vi "Commutator_close.vi"(1 "VISA in":T1) -> (0 "Error out":errorcluster)   [LabVIEW 2011]
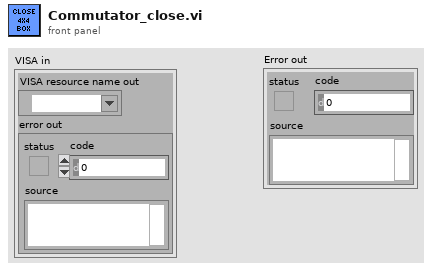
[diagram p1: front panel]
types:
  T1 = cluster{"VISA resource name out":refnum<visa-resource-name>, "error out":errorcluster}
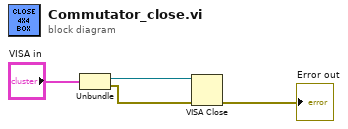
[diagram p0: block diagram]
diagram:
  n1 = Unbundle("VISA in") -> ("VISA resource name out"=w3:refnum<visa-resource-name>, "error out"=w2:errorcluster)
  n2 = VISA Close(VISA resource name=w3, error in (no error)=w2) -> (error out=→"Error out":errorcluster)
